vi "Group7.vi"() -> ()   [LabVIEW 2013]
uses:
  Awesome_Statechart.lvsc/StatechartState.ctl
  Awesome_Statechart.lvsc/State.ctl
  <vilib>/myRIO/Instrument Drivers/Onboard IO/DIO/typedefs/DIO Reference.ctl
  <vilib>/myRIO/Common/Instrument Driver Framework/Utilities/typedefs/myRIO Generic Hardware Reference.ctl
  <vilib>/myRIO/Common/Instrument Driver Framework/Utilities/typedefs/Hardware Version Enum.ctl
  <vilib>/myRIO/Common/Instrument Driver Framework/Utilities/typedefs/myRIO v1.0 Reference.ctl
  <vilib>/myRIO/Common/Instrument Driver Framework/Utilities/typedefs/Generic FPGA Reference.ctl
  <vilib>/myRIO/Common/Instrument Driver Framework/myRIO v1.0/DIO/typedefs/DIO Channels List.ctl
  <vilib>/myRIO/Common/Instrument Driver Framework/myRIO v1.0/DIO/typedefs/DIO Channels Enum.ctl
  <vilib>/myRIO/Instrument Drivers/Onboard IO/AI/typedefs/AI Reference.ctl
  <vilib>/myRIO/Common/Instrument Driver Framework/myRIO v1.0/AI/typedefs/AI Channels List.ctl
  <vilib>/myRIO/Common/Instrument Driver Framework/myRIO v1.0/AI/typedefs/AI Channels Enum.ctl
  <vilib>/myRIO/Common/Instrument Driver Framework/Utilities/typedefs/Analog Scaling Constants List.ctl
  <vilib>/myRIO/Common/Instrument Driver Framework/Utilities/typedefs/Analog Scaling Constants.ctl
  <vilib>/myRIO/Instrument Drivers/Onboard IO/PWM/typedefs/PWM Reference.ctl
  <vilib>/myRIO/Common/Instrument Driver Framework/myRIO v1.0/PWM/typedefs/PWM Channels Enum.ctl
  <vilib>/myRIO/Instrument Drivers/Onboard IO/PWM/typedefs/PWM Configuration.ctl
  <vilib>/Platform/TimedLoop/XDataNode/timing_clust.ctl
  <vilib>/Platform/TimedLoop/XDataNode/nitl_modes.ctl
  <vilib>/Platform/TimedLoop/XDataNode/wakeup.ctl
  Awesome_Statechart.lvsc/Inputs.ctl
  Awesome_Statechart.lvsc/CompanionDiagram.vi/38/SC Main.vi
  <vilib>/myRIO/Common/Instrument Driver Framework/myRIO v1.0/PWM/vis/myRIO v1.1 Open PWM.vi
  <vilib>/myRIO/Common/Instrument Driver Framework/myRIO v1.0/AI/vis/myRIO v1.1 Open AI.vi
  <vilib>/myRIO/Common/Instrument Driver Framework/myRIO v1.0/DIO/vis/myRIO v1.1 Open DIO.vi
  Awesome_Statechart.lvsc/CompanionDiagram.vi/38/Upd State.vi
  Awesome_Statechart.lvsc/CompanionDiagram.vi/38/Trans Graph0.vi
  Awesome_Statechart.lvsc/CompanionDiagram.vi/38/EnterGraphCore.vi
  <vilib>/myRIO/Common/Instrument Driver Framework/myRIO v1.0/PWM/vis/myRIO v1.0 Close PWM.vi
  <vilib>/myRIO/Common/Instrument Driver Framework/myRIO v1.0/AI/vis/myRIO v1.0 Close AI.vi
  <vilib>/myRIO/Common/Instrument Driver Framework/myRIO v1.0/DIO/vis/myRIO v1.0 Close DIO.vi
  <vilib>/myRIO/Common/Instrument Driver Framework/Utilities/vis/Validate Channels.vi
  <vilib>/myRIO/Common/Instrument Driver Framework/myRIO v1.0/PWM/vis/myRIO v1.0 Reserve PWM.vi
  <vilib>/myRIO/Common/Instrument Driver Framework/myRIO v1.0/AI/vis/myRIO v1.0 Reserve AI.vi
  <vilib>/myRIO/Common/Instrument Driver Framework/myRIO v1.0/DIO/vis/myRIO v1.0 Reserve DIO.vi
  Awesome_Statechart.lvsc/CompanionDiagram.vi/38/Trans Graph1.vi
  <vilib>/myRIO/Common/Instrument Driver Framework/myRIO v1.0/PWM/vis/myRIO v1.0 Unreserve PWM.vi
  <vilib>/myRIO/Common/Instrument Driver Framework/myRIO v1.0/AI/vis/myRIO v1.0 Unreserve AI.vi
  <vilib>/myRIO/Common/Instrument Driver Framework/myRIO v1.0/DIO/vis/myRIO v1.0 Unreserve DIO.vi
  <vilib>/myRIO/Common/Instrument Driver Framework/myRIO v1.0/PWM/vis/myRIO v1.0 Build MUX Configuration PWM.vi
  <vilib>/myRIO/Common/Instrument Driver Framework/myRIO v1.0/Resource Manager/vis/myRIO v1.0 Reserve Channel List.vi
  <vilib>/myRIO/Common/Instrument Driver Framework/myRIO v1.0/AI/vis/myRIO v1.0 Build MUX Configuration AI.vi
  <vilib>/myRIO/Common/Instrument Driver Framework/myRIO v1.0/DIO/vis/myRIO v1.0 Build MUX Configuration DIO.vi
  Awesome_Statechart.lvsc/CompanionDiagram.vi/38/Trans Graph2.vi
  <vilib>/myRIO/Common/Instrument Driver Framework/myRIO v1.0/Resource Manager/vis/myRIO v1.0 Unreserve Channel List.vi
  <vilib>/myRIO/Common/Instrument Driver Framework/myRIO v1.0/Resource Manager/vis/myRIO v1.0 Create Configuration List.vi
  <vilib>/myRIO/Common/Instrument Driver Framework/myRIO v1.0/Resource Manager/vis/myRIO v1.0 Reserve Channel.vi
  <vilib>/myRIO/Common/Instrument Driver Framework/myRIO v1.0/Resource Manager/vis/myRIO v1.0 Unreserve Channel.vi
  <vilib>/myRIO/Common/Instrument Driver Framework/myRIO v1.0/Resource Manager/vis/myRIO v1.0 Build Mutex Name.vi
  <vilib>/FPGAPlugInAG/myRIO-1900/niLvFpga_Open_myRIO-1900.vi
  <vilib>/rvi/interface/common/dynamic/niFpgaDynamicAddResources.vi
  <vilib>/myRIO/Common/Instrument Driver Framework/Utilities/vis/FPGA Ref Manager.vi
  <vilib>/Utility/error.llb/Error Cluster From Error Code.vi
  <vilib>/rvi/interface/common/niFpgaWaitOnOcc.vi
  <vilib>/myRIO/Common/Instrument Driver Framework/myRIO v1.0/myRIO v1.1 Open.vi
  <vilib>/Utility/VariantDataType/GetNumericInfo.vi
  <vilib>/myRIO/Common/Instrument Driver Framework/Utilities/vis/IO Manager.vi
  <vilib>/myRIO/Common/Instrument Driver Framework/Utilities/vis/Configuration Manager.vi
  <vilib>/myRIO/Common/Instrument Driver Framework/myRIO v1.0/Resource Manager/vis/myRIO v1.0 Configure IO.vi
  <vilib>/myRIO/Common/Instrument Driver Framework/myRIO v1.0/myRIO v1.0 Close.vi
  <vilib>/myRIO/Common/Instrument Driver Framework/myRIO v1.0/AI/vis/myRIO v1.0 Get Scaling Constants AI.vi
  <vilib>/myRIO/Common/Instrument Driver Framework/myRIO v1.0/DIO/vis/myRIO v1.0 Read DIO.vi
  <vilib>/myRIO/Common/Instrument Driver Framework/myRIO v1.0/DIO/vis/myRIO v1.0 Write DIO.vi
  <vilib>/myRIO/Common/Instrument Driver Framework/myRIO v1.0/PWM/vis/myRIO v1.0 Write PWM.vi
  <vilib>/myRIO/Common/Instrument Driver Framework/myRIO v1.0/AI/vis/myRIO v1.0 Read AI.vi
  Awesome_Statechart.lvsc/CompanionDiagram.vi
  <vilib>/rvi/errors/niLvFpgaAdjustHostInterfaceError.vi
  <vilib>/myRIO/Common/Instrument Driver Framework/myRIO v1.0/DIO/vis/myRIO v1.0 Shutdown DIO.vi
  <vilib>/myRIO/Common/Instrument Driver Framework/myRIO v1.0/PWM/vis/myRIO v1.0 Shutdown PWM.vi
  <vilib>/FPGAPlugInAG/Dynamic/niLvFpga_Close_Dynamic.vi
  <vilib>/rvi/interface/nirviOpenFPGA/nirviOpenFPGA.xnode
  FPGA Bitfiles/MAE162Labs_FPGATarget_myRIO-1900Custom_wGhQFU+VMJc.lvbitx
  <vilib>/rvi/interface/nirviMethod/nirviMethod.xnode
  <vilib>/Platform/TimedLoop/XDataNode/XDataNode.xnode
  Awesome_Statechart.lvsc/Trigger.ctl
  <vilib>/Statechart/Infrastructure/RTStatechart/RunTime SCN.xnode
  Awesome_Statechart.lvsc/Outputs.ctl
  Awesome_Statechart.lvsc
  <vilib>/rvi/interface/nirviCloseFPGA/nirviCloseFPGA.xnode
  <vilib>/Platform/TimedLoop/XDataNode/XDNodeRunTimeDep.lvlib
  <vilib>/rvi/interface/nirviMethod/StockFPGA_InlinedMethodWaitForSingleIRQ.vi
  <vilib>/FPGAPlugInAG/Dynamic/niLvFpga_WaitOnIrq_Dynamic.vi
  <vilib>/FPGAPlugInAG/Dynamic/niLvFpga_AcknowledgeIrq_Dynamic.vi
  <vilib>/myRIO/Instrument Drivers/Utilities/Utilities.lvlib
  <vilib>/myRIO/Instrument Drivers/Onboard IO/DIO/DIO.lvlib
  <vilib>/myRIO/Instrument Drivers/Onboard IO/AI/AI.lvlib
  <vilib>/myRIO/Instrument Drivers/Onboard IO/PWM/PWM.lvlib
panel:
  in  "Pulse Width":dbl=2280.0
  out "Left Duty Cycle":dbl(graph)
  out "Right Duty Cycle":dbl(graph)
  in  "moving up ramp gains":cluster{"Kp":dbl, "Kd":dbl, "Ki":dbl, "Ts":dbl}={"Kp"=0.01, "Kd"=0.0, "Ki"=0.008, "Ts"=0.01}
  out "duty 2":dbl=0.012080000000000046
  in  "Gain Mode 2":dbl=2.5
  out "PID Output 2":dbl=0.004832000000000019
  out "L_DC 2":dbl=-0.38308
  out "R_DC 2":dbl=-0.41692000000000007
  in  "Reverse?":bool
  in  "Default_Speed":dbl=0.4
  in  "On Ramp?":bool
  out "WindUp Servo":i16=1525
  out "R_DC":dbl=0.06510400000000012
  out "L_DC":dbl=-0.06510400000000012
  out "Moving Up Ramp?":bool
  out "Finding Entrance?":bool
  out "PID Output":dbl=0.03272000000000006
  out "R_DC_STATE":dbl
  out "L_DC_STATE":dbl
  out "duty":dbl=0.06544000000000012
  in  "Gain Mode 1":dbl=2.0
  in  "moving down ramp gainz":cluster{"Kp":dbl, "Kd":dbl, "Ki":dbl, "Ts":dbl}={"Kp"=0.02, "Kd"=0.0, "Ki"=0.016, "Ts"=0.01}
  out "Mode":i16=3
  in  "BLACK BOX GRAPH":enum32{"Page 1", "Page 2", "Page 3"}(tab)=enum."Page 2"
  out "Black Box":T1(graph)
  out "Black Box Array":dbl[][](array[numeric])
  out "Array":bool[](array[boolean])
  out "Button Num":u32
  in  "ON":bool
  in  "OFF":bool
  out "Active States":T2=[enum."On", enum."On\\Region\\Running"]
  out "Front Right":dbl=6.1
  out "Front Left":dbl=7.5
  out "Back Right":dbl=7.6
  out "Center":dbl=6.692913385826771
  out "Back Left":dbl=7.9
  out "Finished Late":u16
  out "Emergency Stop":bool=TRUE
  # "1000 to 2000; 1500 max"
  # "Coming Out of Statechart"
  # "2000 max"
  # "800 max"
  # "MOVING DOWN RAMP"
  # "MOVING UP RAMP"
  # "Coming Out of PID"
  # "3rd bin: 2280\n2nd bin: 2150\n1st bin: 1950"
  # "After Calculations"
  # "SENSORS"
  # "gAIN = 2"
  # "MOTORS"
  # "KP=0.02"
  # "moving up:\nKp = 0.01\nki = 0.008\n\nts = 0.01\n\nmoving down:\nkp = 0.02\nki = 0.016\nts = 0.01"
  # "0: Find Entrance\n1: Move Up\n2: Move Down\n3: Default"
  # "SERVOS"
  # "kI = 0.016"
  # "NOTE: Continuous Servo Mid-Point = 1525\nPlatform Servo Mid-Point = 1500"
  # "tS = 0.01"
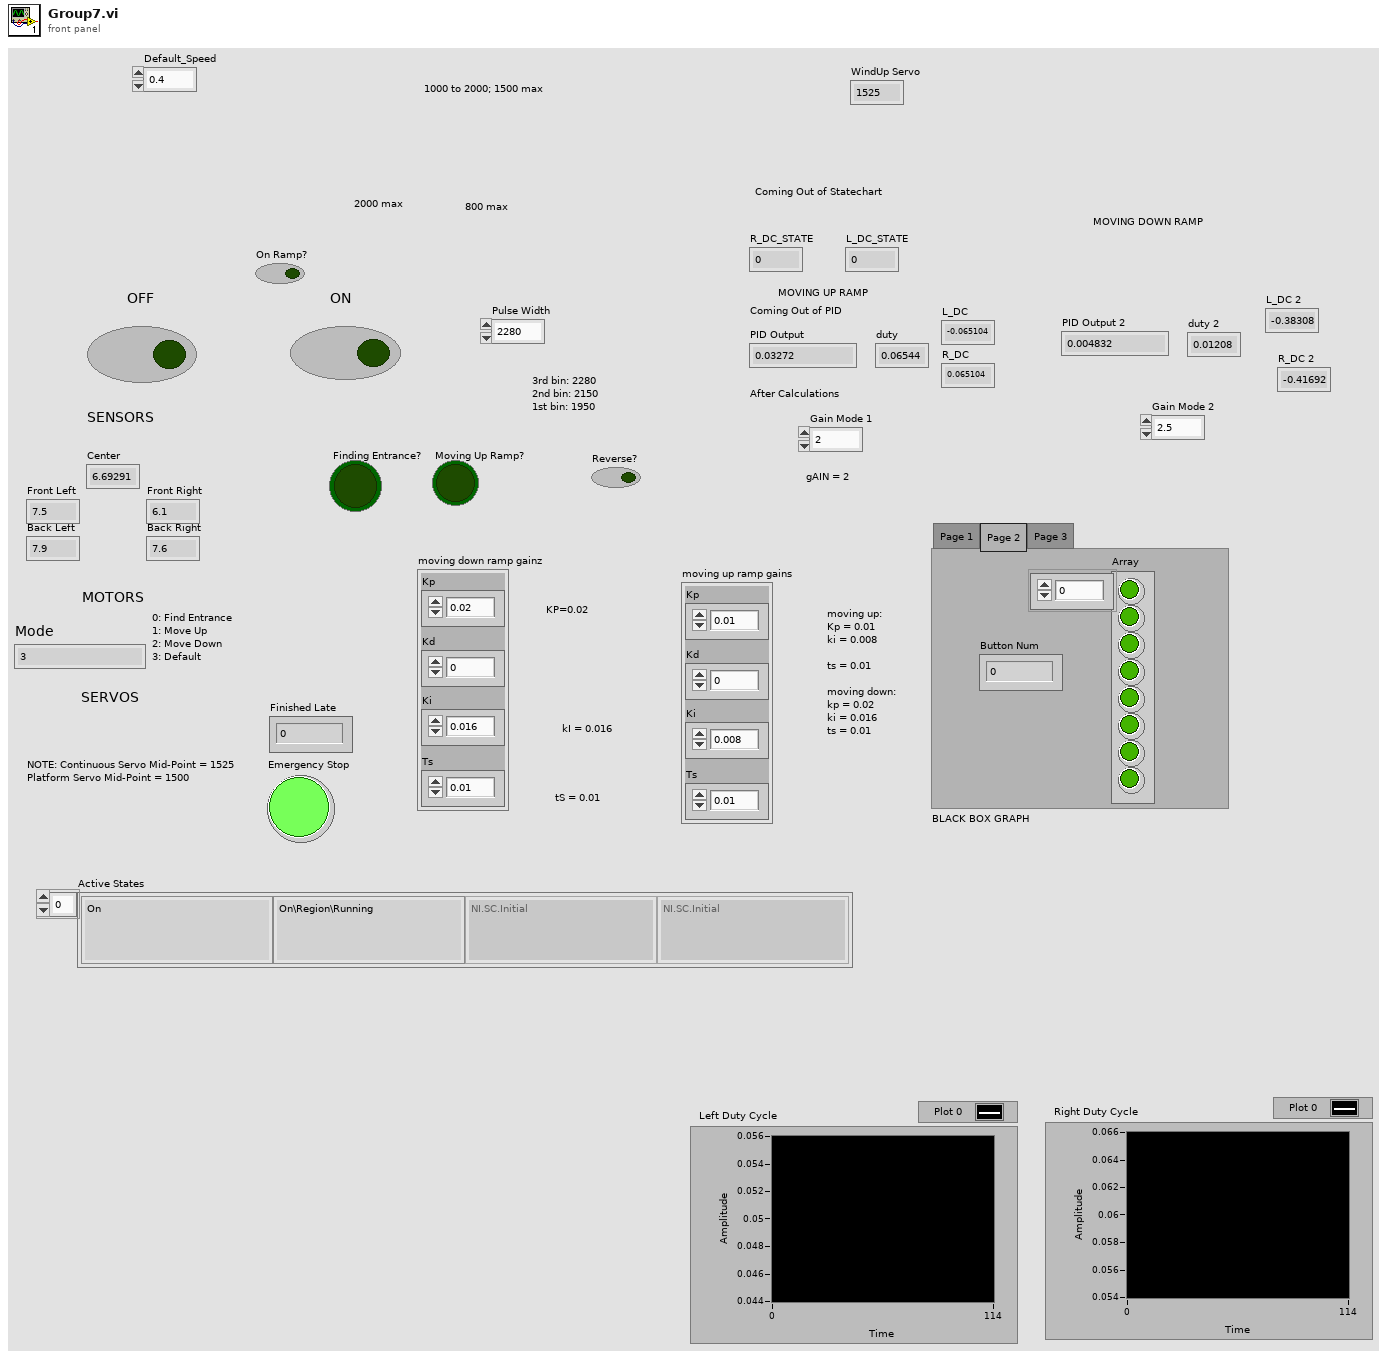
[diagram p1: front panel]
types:
  T1 = cluster{"[0]":dbl, "[1]":dbl, "[2]":dbl, "[3]":dbl, "[4]":dbl, "[5]":dbl, "[6]":dbl, "[7]":dbl}
  T2 = typedef "Awesome_Statechart.lvsc/StatechartState.ctl" = T3[]
  T3 = typedef "Awesome_Statechart.lvsc/State.ctl" = enum16{"NI.SC.Initial", "NI.SC.History", "NI.SC.ShallowHistory", "NI.SC.Terminal", "On", "Off", "On\\Region\\Straighten", "On\\Region\\Wait", "On\\Region\\Fire Cannon", "On\\Region\\Moving Down Ramp", "On\\Region\\Moving Up Ramp", "On\\Region\\Find_Entrance", "On\\Region\\Running", "On\\Region\\Find_Entrance\\Region\\Entrance\nOn\nRight Side", "On\\Region\\Find_Entrance\\Region\\Entrance \nOn\nLeft Side", "On\\Region\\Find_Entrance\\Region\\Turn Right", "On\\Region\\Find_Entrance\\Region\\Turn Left", "On\\Region\\Find_Entrance\\Region\\Go_Straight", "On\\Region\\Find_Entrance\\Region\\Running"}
  T4 = typedef "DIO.lvlib/DIO Reference.ctl" = cluster{"myRIO Reference":T5, "DIO Channels List":T9}
  T5 = typedef "myRIO Generic Hardware Reference.ctl" = cluster{"myRIO Model":T6, "myRIO Hardware Reference":T7}
  T6 = typedef "Hardware Version Enum.ctl" = enum16{"Unknown", "myRIO-1900", "myRIO-1950"}
  T7 = typedef "myRIO v1.0 Reference.ctl" = cluster{"Generic FPGA Reference":T8, "Allow multiple opens":bool}
  T8 = typedef "Generic FPGA Reference.ctl" = refnum<k20>
  T9 = typedef "DIO Channels List.ctl" = T10[]
  T10 = typedef "DIO Channels Enum.ctl" = enum16{"Not Connected", "C/DIO0", "C/DIO1", "C/DIO2", "C/DIO3", "C/DIO4", "C/DIO5", "C/DIO6", "C/DIO7", "A/DIO0", "A/DIO1", "A/DIO2", "A/DIO3", "A/DIO4", "A/DIO5", "A/DIO6", "A/DIO7", "A/DIO8", "A/DIO9", "A/DIO10", "A/DIO11", "A/DIO12", "A/DIO13", "A/DIO14", "A/DIO15", "B/DIO0", "B/DIO1", "B/DIO2", "B/DIO3", "B/DIO4", "B/DIO5", "B/DIO6", "B/DIO7", "B/DIO8", "B/DIO9", "B/DIO10", "B/DIO11", "B/DIO12", "B/DIO13", "B/DIO14", "B/DIO15", "LED0", "LED1", "LED2", "LED3", "Button0"}
  T11 = typedef "AI.lvlib/AI Reference.ctl" = cluster{"myRIO Reference":T5, "AI Channels List":T12, "AI Scaling Constants List":T14}
  T12 = typedef "AI Channels List.ctl" = T13[]
  T13 = typedef "AI Channels Enum.ctl" = enum16{"Not Connected", "AudioIn/Left", "AudioIn/Right", "C/AI0", "C/AI1", "A/AI0", "A/AI1", "A/AI2", "A/AI3", "B/AI0", "B/AI1", "B/AI2", "B/AI3"}
  T14 = typedef "Analog Scaling Constants List.ctl" = T15[]
  T15 = typedef "Analog Scaling Constants.ctl" = cluster{"LSB Weight (Volts)":dbl, "Offset (Volts)":dbl, "Signed?":bool}
  T16 = typedef "PWM.lvlib/PWM Reference.ctl" = cluster{"myRIO Reference":T5, "PWM Channels Enum":T17, "PWM Configuration":T18}
  T17 = typedef "PWM Channels Enum.ctl" = enum16{"Not Connected", "C/PWM0", "C/PWM1", "A/PWM0", "A/PWM1", "A/PWM2", "B/PWM0", "B/PWM1", "B/PWM2"}
  T18 = typedef "PWM.lvlib/PWM Configuration.ctl" = cluster{"Frequency":dbl, "Duty Cycle":dbl}
  T19 = cluster{"Button Ref":T4, "LED Ref":T4, "Front_Right":T11, "Front_Left":T11, "Back_Right":T11, "Front_Center\nBI Ref 1":T11, "Back_Left\nBI Ref 2":T11, "Windup":T16, "Platform_S\nPlatform_S\nContinuous Servo":T16, "Left Motor\nLeft Motor\nright_motor":T16, "Right Motor\nleft_motor":T16}
  T20 = typedef "XDNodeRunTimeDep.lvlib/timing_clust.ctl" = cluster{"Expected End [f-1]":u64, "Actual End [f-1]":u64, "Finished Late? [f-1]":bool, "Expected End [i-1]":u64, "Actual End [i-1]":u64, "Finished Late? [i-1]":bool, "Expected Start [i]":u64, "Actual Start [i]":u64, "Expected Start [f]":u64, "Actual Start [f]":u64, "Source Name":string, "Structure Name":string, "Period":i64, "Deadline":i64, "Offset":i64, "Start":i64, "Priority":i32, "Timeout":i32, "Mode":T21, "Wakeup Reason":T22, "Error":errorcluster, "Source Type":string, "Secondary Source Type":string, "Global End Time":u64, "Global Start Time":u64, "Frame Duration":u64, "Iteration Duration":u64, "Assigned CPU":i32, "I/O Scan Engine Mode":u32}
  T21 = typedef "XDNodeRunTimeDep.lvlib/nitl_modes.ctl" = enum32{"No Change", "Process missed periods, maintain original phase", "Discard missed periods, maintain original phase", "Process missed periods, ignore original phase", "Discard missed periods, ignore original phase"}
  T22 = typedef "XDNodeRunTimeDep.lvlib/wakeup.ctl" = enum32{"Normal", "Aborted", "Asynchronous wakeup", "Timing source error", "Timed loop error", "Timeout"}
  T23 = typedef "Awesome_Statechart.lvsc/Inputs.ctl" = cluster{"On/Set":bool, "Off":bool, "Front_Center ":dbl, "Front_Left":dbl, "Front_Right":dbl, "Back_Left":dbl, "Back_Right":dbl, "Find_Entrance?":bool, "Default_Speed":dbl, "On Ramp?":bool, "Bombs Away!":bool, "Reverse?":bool}
  T24 = typedef "Awesome_Statechart.lvsc/Outputs.ctl" = cluster{"Left_Duty":dbl, "Right_Duty":dbl, "Mode":i16, "Finding Entrance?":bool, "Moving Up Ramp?":bool, "WindUp Servo":i16, "Straighten?":bool, "Platform Servo":dbl}
  T25 = cluster{"[0]":dbl, "[1]":dbl, "[2]":dbl, "[3]":dbl, "[4]":dbl, "[5]":dbl, "[6]":dbl, "[7]":dbl}[]
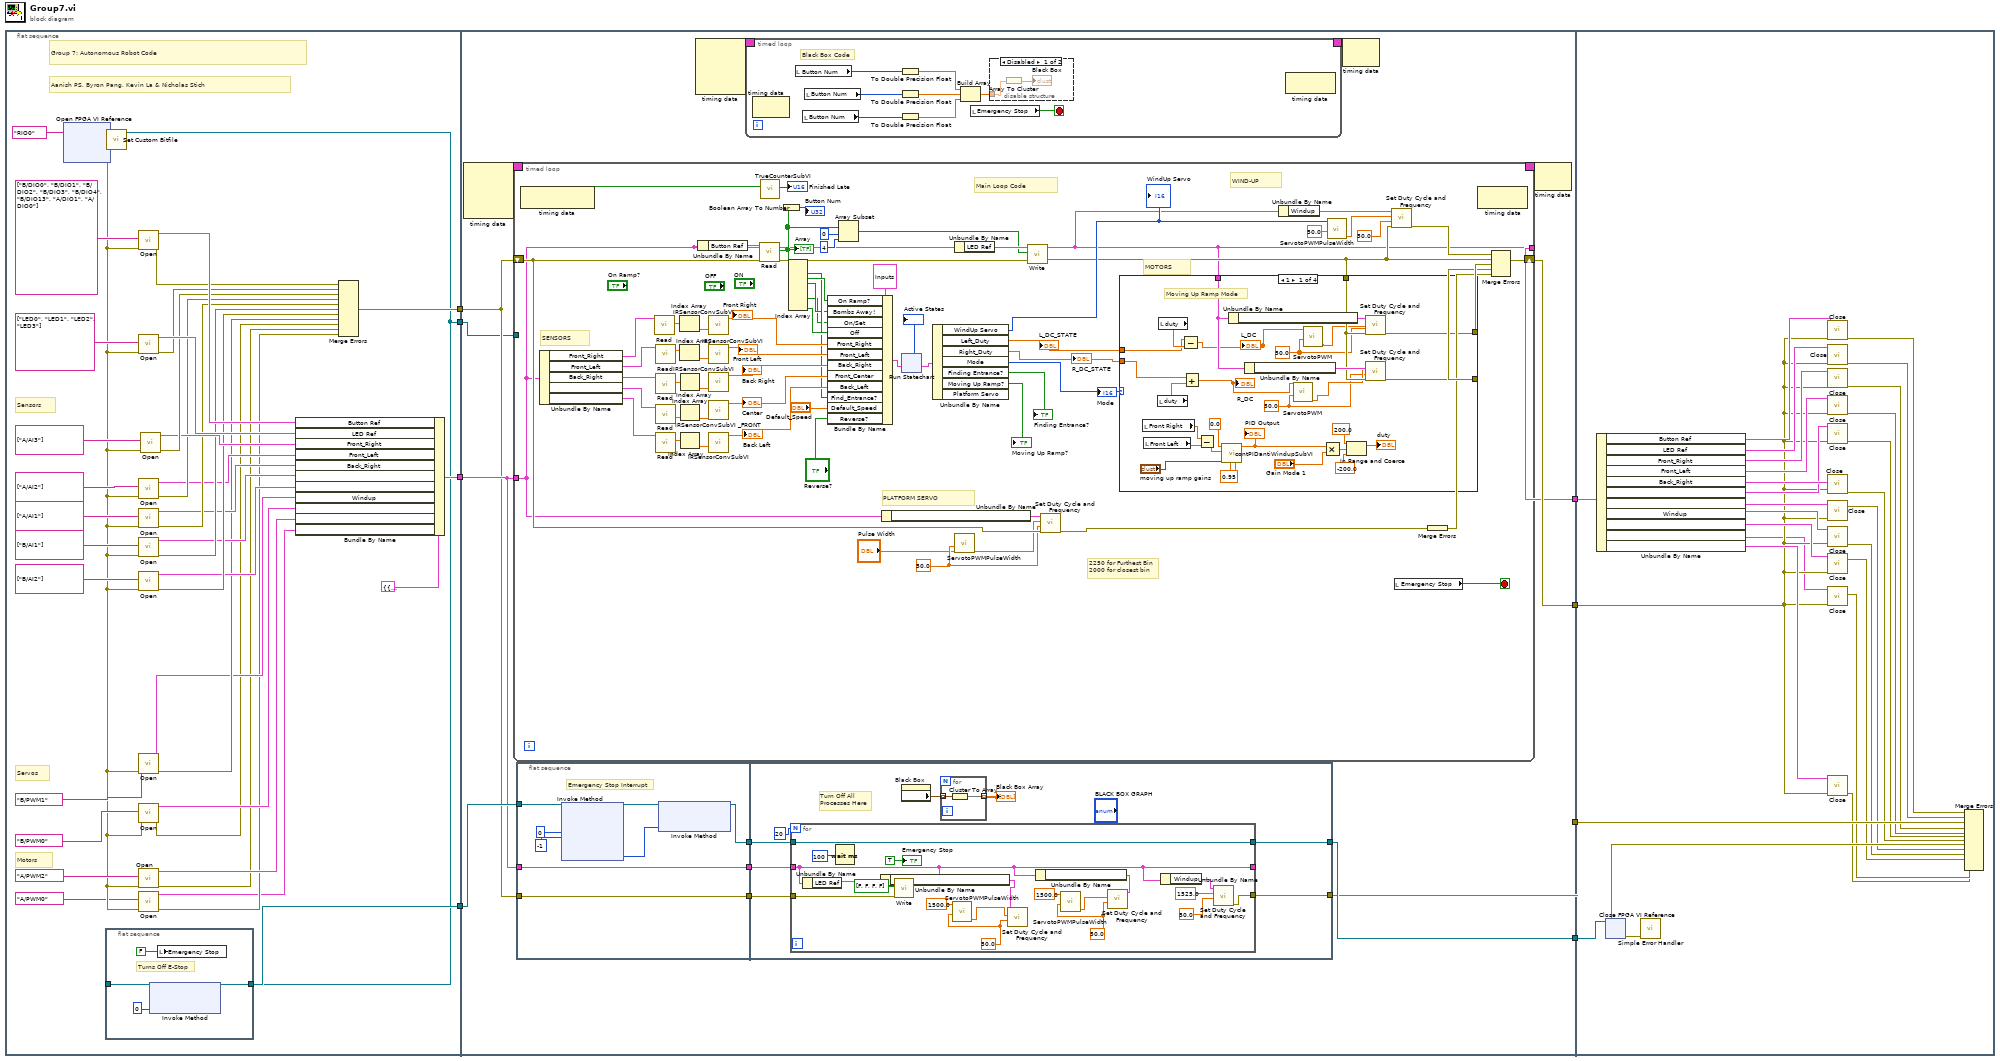
[diagram p0: block diagram]
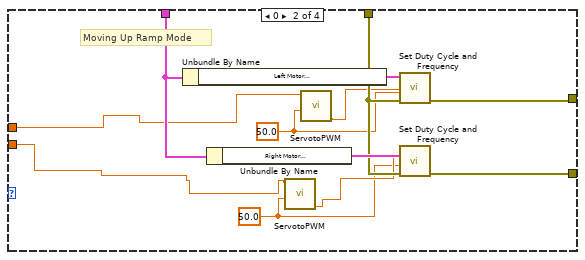
[diagram p3: hidden frame]
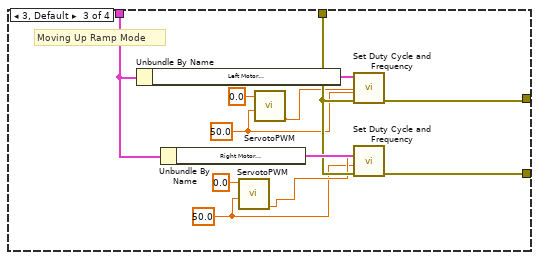
[diagram p4: hidden frame]
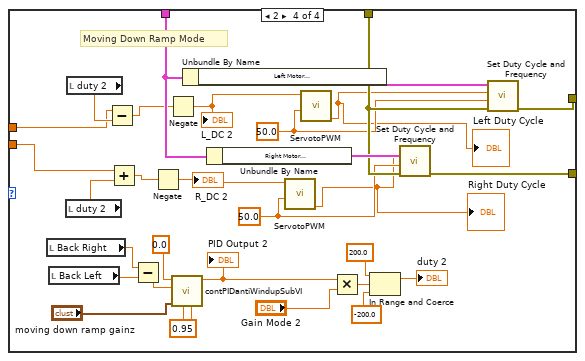
[diagram p5: hidden frame]
diagram:
  n1 = flat-sequence {
    tunnel: [w50] -> w8
    tunnel: [w40] -> w6
    tunnel: [w39] -> w5
    tunnel: [w38] -> w1
    tunnel: [w64] -> w7
    tunnel: w8 -> [w63]
    tunnel: w6 -> [w62]
    tunnel: w5 -> [w59]
    tunnel: [w58] -> w4
    tunnel: [w55] -> w3
    tunnel: [w57] -> w2
    tunnel: w1 -> [w56]
    tunnel: w7 -> [w405]
    tunnel: w4 -> [w379]
    tunnel: w3 -> [w404]
    tunnel: w2 -> [w397]
    frame #0 {
      # "Aanish PS, Byron Pang, Kevin La & Nicholas Stich"
      # "Group 7: Autonomous Robot Code"
      # "Servos"
      # "Motors"
      # "Sensors"
      n2 = xnode "Open FPGA VI Reference"("resource name"=tag "RIO0") -> ("FPGA VI Reference Out"=w49:refnum<k20>, "error out"=w48:errorcluster)  [unwired: 1 in]
      n3 = flat-sequence {
        tunnel: [w52] -> w50
        tunnel: w38 -> [w53]
        frame #0 {
          # "Turns Off E-Stop"
          n4 = xnode "Invoke Method"("FPGA VI Reference In"=w53, "IRQ Number(s)"=0) -> ("FPGA VI Reference Out"=w52:refnum<k20>)  [unwired: 1 in, 1 out]
          n5 = local write "Emergency Stop"(FALSE ("Emergency Stop")) -> ()
        }
      }
      n6 = call <vilib>:"Set Custom Bitfile.vi"("error in (no error)"=w48, "Customized FPGA Reference in"=w49) -> ("error out"=w15:errorcluster, "Customized FPGA Reference out"=w38:refnum<k20>)  [unwired: 8 in]
      n7 = call <vilib>:"Open.vi"("error in (no error)"=w15, "Channel Names"=tag[] ["B/DIO0", "B/DIO1", "B/DIO2", "B/DIO3", "B/DIO4", "B/DIO13", "A/DIO1", "A/DIO0"]) -> ("error out"=w42:errorcluster, "DIO Ref Out"=w44:T4)  [unwired: 8 in]
      n8 = call <vilib>:"Open.vi"("error in (no error)"=w15, "Channel Names"=tag[] ["LED0", "LED1", "LED2", "LED3"]) -> ("error out"=w41:errorcluster, "DIO Ref Out"=w43:T4)  [unwired: 8 in]
      n9 = call <vilib>:"Open.vi"("error in (no error)"=w15, "Channel Names"=tag[] ["A/AI2"]) -> ("error out"=w32:errorcluster, "AI Ref Out"=w26:T11)  [unwired: 8 in]
      n10 = call <vilib>:"Open.vi"("error in (no error)"=w15, "Channel Names"=tag[] ["A/AI1"]) -> ("error out"=w31:errorcluster, "AI Ref Out"=w25:T11)  [unwired: 8 in]
      n11 = call <vilib>:"Open.vi"("error in (no error)"=w15, "Channel Names"=tag[] ["B/AI1"]) -> ("error out"=w29:errorcluster, "AI Ref Out"=w24:T11)  [unwired: 8 in]
      n12 = call <vilib>:"Open.vi"("error in (no error)"=w15, "Channel Names"=tag[] ["B/AI2"]) -> ("error out"=w27:errorcluster, "AI Ref Out"=w23:T11)  [unwired: 8 in]
      n13 = call <vilib>:"Open.vi"("error in (no error)"=w15, "Channel Name"=tag "B/PWM1") -> ("error out"=w21:errorcluster, "PWM Ref Out"=w20:T16)  [unwired: 8 in]
      n14 = call <vilib>:"Open.vi"("error in (no error)"=w15, "Channel Name"=tag "B/PWM0") -> ("error out"=w11:errorcluster, "PWM Ref Out"=w18:T16)  [unwired: 8 in]
      n15 = call <vilib>:"Open.vi"("error in (no error)"=w15, "Channel Name"=tag "A/PWM2") -> ("error out"=w10:errorcluster, "PWM Ref Out"=w16:T16)  [unwired: 8 in]
      n16 = call <vilib>:"Open.vi"("error in (no error)"=w15, "Channel Name"=tag "A/PWM0") -> ("error out"=w13:errorcluster, "PWM Ref Out"=w12:T16)  [unwired: 8 in]
      n17 = call <vilib>:"Open.vi"("error in (no error)"=w15, "Channel Names"=tag[] ["A/AI3"]) -> ("error out"=w37:errorcluster, "AI Ref Out"=w36:T11)  [unwired: 8 in]
      n18 = Bundle By Name(cluster=T19 {"Button Ref"={"myRIO Reference"={"myRIO Model"=enum."Unknown", "myRIO Hardware Reference"={"Generic FPGA Reference"=refnum, "Allow multiple opens"=FALSE}}, "DIO Channels List"=[]}, "LED Ref"={"myRIO Reference"={"myRIO Model"=enum."Unknown", "myRIO Hardware Reference"={"Generic FPGA Reference"=refnum, "Allow multiple opens"=FALSE}}, "DIO Channels List"=[]}, "Front_Right"={"myRIO Reference"={"myRIO Model"=enum."Unknown", "myRIO Hardware Reference"={"Generic FPGA Reference"=refnum, "Allow multiple opens"=FALSE}}, "AI Channels List"=[], "AI Scaling Constants List"=[]}, "Front_Left"={"myRIO Reference"={"myRIO Model"=enum."Unknown", "myRIO Hardware Reference"={"Generic FPGA Reference"=refnum, "Allow multiple opens"=FALSE}}, "AI Channels List"=[], "AI Scaling Constants List"=[]}, "Back_Right"={"myRIO Reference"={"myRIO Model"=enum."Unknown", "myRIO Hardware Reference"={"Generic FPGA Reference"=refnum, "Allow multiple opens"=FALSE}}, "AI Channels List"=[], "AI Scaling Constants List"=[]}, "Front_Center\nBI Ref 1"={"myRIO Reference"={"myRIO Model"=enum."Unknown", "myRIO Hardware Reference"={"Generic FPGA Reference"=refnum, "Allow multiple opens"=FALSE}}, "AI Channels List"=[], "AI Scaling Constants List"=[]}, "Back_Left\nBI Ref 2"={"myRIO Reference"={"myRIO Model"=enum."Unknown", "myRIO Hardware Reference"={"Generic FPGA Reference"=refnum, "Allow multiple opens"=FALSE}}, "AI Channels List"=[], "AI Scaling Constants List"=[]}, "Windup"={"myRIO Reference"={"myRIO Model"=enum."Unknown", "myRIO Hardware Reference"={"Generic FPGA Reference"=refnum, "Allow multiple opens"=FALSE}}, "PWM Channels Enum"=enum."Not Connected", "PWM Configuration"={"Frequency"=0.0, "Duty Cycle"=0.0}}, "Platform_S\nPlatform_S\nContinuous Servo"={"myRIO Reference"={"myRIO Model"=enum."Unknown", "myRIO Hardware Reference"={"Generic FPGA Reference"=refnum, "Allow multiple opens"=FALSE}}, "PWM Channels Enum"=enum."Not Connected", "PWM Configuration"={"Frequency"=0.0, "Duty Cycle"=0.0}}, "Left Motor\nLeft Motor\nright_motor"={"myRIO Reference"={"myRIO Model"=enum."Unknown", "myRIO Hardware Reference"={"Generic FPGA Reference"=refnum, "Allow multiple opens"=FALSE}}, "PWM Channels Enum"=enum."Not Connected", "PWM Configuration"={"Frequency"=0.0, "Duty Cycle"=0.0}}, "Right Motor\nleft_motor"={"myRIO Reference"={"myRIO Model"=enum."Unknown", "myRIO Hardware Reference"={"Generic FPGA Reference"=refnum, "Allow multiple opens"=FALSE}}, "PWM Channels Enum"=enum."Not Connected", "PWM Configuration"={"Frequency"=0.0, "Duty Cycle"=0.0}}}, "Button Ref"=w44, "LED Ref"=w43, "Front_Right"=w36, "Front_Left"=w26, "Back_Right"=w25, "Front_Center\nBI Ref 1"=w24, "Back_Left\nBI Ref 2"=w23, "Windup"=w20, "Platform_S\nPlatform_S\nContinuous Servo"=w18, "Left Motor\nLeft Motor\nright_motor"=w16, "Right Motor\nleft_motor"=w12) -> (w40:T19)
      n19 = Merge Errors(w42, w41, w37, w32, w31, w29, w27, w21, w11, w10, w13) -> (w39:errorcluster)
    }
    frame #1 {
      n20 = node-c288() -> (w69:T20)  [unwired: 4 in]
      n21 = timed-loop {
        timing: w69 -> [_]
        timing-out: [_] -> w68
        tunnel: w62 -> [w134]
        tunnel: [w134] -> w55
        shift-right: [w161] -> w58
        shift-left: w59 -> [w139]
        tunnel: w56 -> [_]
        stop <- w185 stop-if-true
        w124 = 50.0 ("Frequency (Hz)")
        # "PLATFORM SERVO"
        # "MOTORS"
        # "2250 for Furthest Bin\n2000 for closest bin"
        # "WIND-UP"
        # "SENSORS"
        # "Main Loop Code"
        n22 = node-c288() -> (w183:bool)  [unwired: 1 in]
        n23 = Unbundle By Name(w134) -> ("Front_Right"=w162:T11, "Front_Left"=w163:T11, "Back_Right"=w156:T11, "Front_Center\nBI Ref 1"=w164:T11, "Back_Left\nBI Ref 2"=w165:T11)
        n24 = call <vilib>:"Read.vi"("AI Ref In"=w162) -> ("Values"=w175:dbl[])  [unwired: 8 in, 2 out]
        n25 = call <vilib>:"Read.vi"("AI Ref In"=w163) -> ("Values"=w174:dbl[])  [unwired: 8 in, 2 out]
        n26 = call <vilib>:"Read.vi"("AI Ref In"=w156) -> ("Values"=w173:dbl[])  [unwired: 8 in, 2 out]
        n27 = call <vilib>:"Read.vi"("AI Ref In"=w164) -> ("Values"=w172:dbl[])  [unwired: 8 in, 2 out]
        n28 = call <vilib>:"Read.vi"("AI Ref In"=w165) -> ("Values"=w171:dbl[])  [unwired: 8 in, 2 out]
        n29 = Index Array(array=w175) -> (element=w170:dbl)  [unwired: 1 in]
        n30 = Index Array(array=w174) -> (element=w167:dbl)  [unwired: 1 in]
        n31 = Index Array(array=w173) -> (element=w168:dbl)  [unwired: 1 in]
        n32 = Index Array(array=w172) -> (element=w166:dbl)  [unwired: 1 in]
        n33 = Index Array(array=w171) -> (element=w169:dbl)  [unwired: 1 in]
        n34 = Unbundle By Name(w134) -> ("Button Ref"=w179:T4)
        n35 = call "IRSensorConvSubVI.vi"("Infrared Sensor Reading"=w170) -> ("Sensor Data"=w152:dbl)  [unwired: 10 in]
        "Front Right" <- w152
        n36 = call "IRSensorConvSubVI.vi"("Infrared Sensor Reading"=w167) -> ("Sensor Data"=w149:dbl)  [unwired: 10 in]
        "Front Left" <- w149
        n37 = call "IRSensorConvSubVI.vi"("Infrared Sensor Reading"=w168) -> ("Sensor Data"=w155:dbl)  [unwired: 10 in]
        "Back Right" <- w155
        n38 = call "IRSensorConvSubVI _FRONT.vi"("Infrared Sensor Reading"=w166) -> ("Sensor Data"=w154:dbl)  [unwired: 10 in]
        "Center" <- w154
        n39 = call "IRSensorConvSubVI.vi"("Infrared Sensor Reading"=w169) -> ("Sensor Data"=w153:dbl)  [unwired: 10 in]
        "Back Left" <- w153
        n40 = call <vilib>:"Read.vi"("error in (no error)"=w139, "DIO Ref In"=w179) -> ("error out"=w178:errorcluster, "Values"=w145:bool[])  [unwired: 7 in, 1 out]
        "Array" <- w145
        n41 = call "TrueCounterSubVI.vi"("True?"=w183) -> ("True Count"=→"Finished Late":u16)  [unwired: 9 in]
        n42 = Boolean Array To Number(Boolean array=w145) -> (number=→"Button Num":u32)
        n43 = Index Array(array=w145) -> (element #1=w128:bool, element #2=w132:bool, element #3=w127:bool, element #6=w126:bool, element #8=w129:bool)  [unwired: 8 in, 3 out]
        n44 = Bundle By Name(cluster=T23 {"On/Set"=FALSE, "Off"=FALSE, "Front_Center "=0.0, "Front_Left"=0.0, "Front_Right"=0.0, "Back_Left"=0.0, "Back_Right"=0.0, "Find_Entrance?"=FALSE, "Default_Speed"=0.0, "On Ramp?"=FALSE, "Bombs Away!"=FALSE, "Reverse?"=FALSE} ("Inputs"), "On Ramp?"=w132, "Bombs Away!"=w127, "On/Set"=w126, "Off"=w129, "Front_Right"=w152, "Front_Left"=w149, "Back_Right"=w155, "Front_Center"=w154, "Back_Left"=w153, "Find_Entrance?"=w128, "Default_Speed"="Default_Speed", "Reverse?"="Reverse?") -> (w159:T23)
        n45 = Array Subset(array=w145, index=0, length=4) -> (w176:bool[])
        n46 = Unbundle By Name(w134) -> ("Platform_S\nPlatform_S\nContinuous Servo"=w123:T16)
        n47 = xnode "Run Statechart"("Inputs"=w159) -> ("Outputs"=w157:T24, "Active States"=→"Active States":T2)  [unwired: 2 in, 1 out]
        n48 = Unbundle By Name(w157) -> ("WindUp Servo"=w142:i16, "Left_Duty"=w147:dbl, "Right_Duty"=w148:dbl, "Mode"=w146:i16, "Finding Entrance?"=→"Finding Entrance?":bool, "Moving Up Ramp?"=→"Moving Up Ramp?":bool)  [unwired: 1 out]
        "Mode" <- w146
        "L_DC_STATE" <- w147
        "R_DC_STATE" <- w148
        "WindUp Servo" <- w142
        n49 = Unbundle By Name(w134) -> ("LED Ref"=w177:T4)
        n50 = call "ServotoPWMPulseWidth.vi"("freq [Hz]"=w124, "Pulse Width"="Pulse Width") -> ("Duty Cycle"=w122:dbl)  [unwired: 6 in, 2 out]
        n51 = call <vilib>:"Write.vi"("error in (no error)"=w178, "Values"=w176, "DIO Ref In"=w177) -> ("error out"=w140:errorcluster)  [unwired: 6 in, 1 out]
        n52 = call <vilib>:"Set Duty Cycle and Frequency.vi"("error in (no error)"=w139, "Frequency (Hz)"=w124, "Duty Cycle (0-1)"=w122, "PWM Ref In"=w123) -> ("error out"=w125:errorcluster)  [unwired: 5 in, 1 out]
        n53 = case shown="1" w146 {
          tunnel: w134 -> [w213 w225 w237 w267]
          tunnel: [w210 w222 w234 w264] -> w151
          tunnel: [w209 w221 w233 w263] -> w150
          tunnel: w148 -> [w195 w214 _ w249]
          tunnel: w147 -> [w193 w215 _ w247]
          tunnel: w140 -> [w198 w220 w232 w252]
          frame 1 {
            w200 = 0.95 ("Saturation U")
            w189 = 50.0 ("freq [Hz]")
            w191 = 50.0 ("freq [Hz]")
            # "Moving Up Ramp Mode"
            n54 = local read "Front Right"() -> (w207:dbl)
            n55 = local read "Front Left"() -> (w205:dbl)
            n56 = local read "duty"() -> (w196:dbl)
            n57 = local read "duty"() -> (w194:dbl)
            n58 = Subtract(x=w193, y=w194) -> (x-y=w187:dbl)
            "L_DC" <- w187
            n59 = Add(x=w195, y=w196) -> (x+y=w188:dbl)
            "R_DC" <- w188
            n60 = Subtract(x=w207, y=w205) -> (x-y=w206:dbl)
            n61 = call "contPIDantiWindupSubVI.vi"("Saturation M"=w200, "Saturation U"=w200, "PID Gains"="moving up ramp gains", "Position"=w206, "Reference"=0.0) -> ("control"=w197:dbl)  [unwired: 6 in]
            "PID Output" <- w197
            n62 = Unbundle By Name(w213) -> ("Left Motor\nLeft Motor\nright_motor"=w212:T16)
            n63 = Unbundle By Name(w213) -> ("Right Motor\nleft_motor"=w211:T16)
            n64 = call "ServotoPWM.vi"("freq [Hz]"=w189, "Duty In"=w188) -> ("Duty Cycle"=w190:dbl)  [unwired: 6 in, 2 out]
            n65 = call "ServotoPWM.vi"("freq [Hz]"=w191, "Duty In"=w187) -> ("Duty Cycle"=w192:dbl)  [unwired: 6 in, 2 out]
            n66 = Multiply(x=w197, y="Gain Mode 1") -> (x*y=w204:dbl)
            n67 = In Range and Coerce(upper limit=200.0, x=w204, lower limit=-200.0) -> (coerced(x)=→"duty":dbl)  [unwired: 1 out]
            n68 = call <vilib>:"Set Duty Cycle and Frequency.vi"("error in (no error)"=w198, "Frequency (Hz)"=w191, "Duty Cycle (0-1)"=w192, "PWM Ref In"=w212) -> ("error out"=w210:errorcluster)  [unwired: 5 in, 1 out]
            n69 = call <vilib>:"Set Duty Cycle and Frequency.vi"("error in (no error)"=w198, "Frequency (Hz)"=w189, "Duty Cycle (0-1)"=w190, "PWM Ref In"=w211) -> ("error out"=w209:errorcluster)  [unwired: 5 in, 1 out]
          }
          frame 0 {
            w216 = 50.0 ("freq [Hz]")
            w218 = 50.0 ("freq [Hz]")
            # "Moving Up Ramp Mode"
            n70 = Unbundle By Name(w225) -> ("Left Motor\nLeft Motor\nright_motor"=w224:T16)
            n71 = Unbundle By Name(w225) -> ("Right Motor\nleft_motor"=w223:T16)
            n72 = call "ServotoPWM.vi"("freq [Hz]"=w216, "Duty In"=w214) -> ("Duty Cycle"=w217:dbl)  [unwired: 6 in, 2 out]
            n73 = call "ServotoPWM.vi"("freq [Hz]"=w218, "Duty In"=w215) -> ("Duty Cycle"=w219:dbl)  [unwired: 6 in, 2 out]
            n74 = call <vilib>:"Set Duty Cycle and Frequency.vi"("error in (no error)"=w220, "Frequency (Hz)"=w218, "Duty Cycle (0-1)"=w219, "PWM Ref In"=w224) -> ("error out"=w222:errorcluster)  [unwired: 5 in, 1 out]
            n75 = call <vilib>:"Set Duty Cycle and Frequency.vi"("error in (no error)"=w220, "Frequency (Hz)"=w216, "Duty Cycle (0-1)"=w217, "PWM Ref In"=w223) -> ("error out"=w221:errorcluster)  [unwired: 5 in, 1 out]
          }
          frame 3, Default {
            w228 = 50.0 ("freq [Hz]")
            w230 = 50.0 ("freq [Hz]")
            # "Moving Up Ramp Mode"
            n76 = Unbundle By Name(w237) -> ("Left Motor\nLeft Motor\nright_motor"=w236:T16)
            n77 = Unbundle By Name(w237) -> ("Right Motor\nleft_motor"=w235:T16)
            n78 = call "ServotoPWM.vi"("freq [Hz]"=w228, "Duty In"=0.0) -> ("Duty Cycle"=w229:dbl)  [unwired: 6 in, 2 out]
            n79 = call "ServotoPWM.vi"("freq [Hz]"=w230, "Duty In"=0.0) -> ("Duty Cycle"=w231:dbl)  [unwired: 6 in, 2 out]
            n80 = call <vilib>:"Set Duty Cycle and Frequency.vi"("error in (no error)"=w232, "Frequency (Hz)"=w230, "Duty Cycle (0-1)"=w231, "PWM Ref In"=w236) -> ("error out"=w234:errorcluster)  [unwired: 5 in, 1 out]
            n81 = call <vilib>:"Set Duty Cycle and Frequency.vi"("error in (no error)"=w232, "Frequency (Hz)"=w228, "Duty Cycle (0-1)"=w229, "PWM Ref In"=w235) -> ("error out"=w233:errorcluster)  [unwired: 5 in, 1 out]
          }
          frame 2 {
            w254 = 0.95 ("Saturation U")
            w245 = 50.0 ("freq [Hz]")
            w246 = 50.0 ("freq [Hz]")
            # "Moving Down Ramp Mode"
            n82 = local read "Back Right"() -> (w261:dbl)
            n83 = local read "Back Left"() -> (w259:dbl)
            n84 = local read "duty 2"() -> (w250:dbl)
            n85 = local read "duty 2"() -> (w248:dbl)
            n86 = Subtract(x=w247, y=w248) -> (x-y=w243:dbl)
            n87 = Add(x=w249, y=w250) -> (x+y=w242:dbl)
            n88 = Subtract(x=w261, y=w259) -> (x-y=w260:dbl)
            n89 = Negate(x=w242) -> (-x=w241:dbl)
            "R_DC 2" <- w241
            n90 = Negate(x=w243) -> (-x=w244:dbl)
            "L_DC 2" <- w244
            n91 = call "contPIDantiWindupSubVI.vi"("Saturation M"=w254, "Saturation U"=w254, "PID Gains"="moving down ramp gainz", "Position"=w260, "Reference"=0.0) -> ("control"=w251:dbl)  [unwired: 6 in]
            "PID Output 2" <- w251
            n92 = Unbundle By Name(w267) -> ("Left Motor\nLeft Motor\nright_motor"=w266:T16)
            n93 = Unbundle By Name(w267) -> ("Right Motor\nleft_motor"=w265:T16)
            n94 = call "ServotoPWM.vi"("freq [Hz]"=w245, "Duty In"=w241) -> ("Duty Cycle"=w239:dbl)  [unwired: 6 in, 2 out]
            "Right Duty Cycle" <- w239
            n95 = call "ServotoPWM.vi"("freq [Hz]"=w246, "Duty In"=w244) -> ("Duty Cycle"=w238:dbl)  [unwired: 6 in, 2 out]
            "Left Duty Cycle" <- w238
            n96 = Multiply(x=w251, y="Gain Mode 2") -> (x*y=w258:dbl)
            n97 = In Range and Coerce(upper limit=200.0, x=w258, lower limit=-200.0) -> (coerced(x)=→"duty 2":dbl)  [unwired: 1 out]
            n98 = call <vilib>:"Set Duty Cycle and Frequency.vi"("error in (no error)"=w252, "Frequency (Hz)"=w245, "Duty Cycle (0-1)"=w239, "PWM Ref In"=w265) -> ("error out"=w263:errorcluster)  [unwired: 5 in, 1 out]
            n99 = call <vilib>:"Set Duty Cycle and Frequency.vi"("error in (no error)"=w252, "Frequency (Hz)"=w246, "Duty Cycle (0-1)"=w238, "PWM Ref In"=w266) -> ("error out"=w264:errorcluster)  [unwired: 5 in, 1 out]
          }
        }
        n100 = Unbundle By Name(w134) -> ("Windup"=w137:T16)
        n101 = call "ServotoPWMPulseWidth.vi"("freq [Hz]"=50.0, "Pulse Width"=w142) -> ("Duty Cycle"=w135:dbl)  [unwired: 6 in, 2 out]
        n102 = call <vilib>:"Set Duty Cycle and Frequency.vi"("error in (no error)"=w140, "Frequency (Hz)"=50.0, "Duty Cycle (0-1)"=w135, "PWM Ref In"=w137) -> ("error out"=w141:errorcluster)  [unwired: 5 in, 1 out]
        n103 = local read "Emergency Stop"() -> (w185:bool)
        n104 = Merge Errors(w125) -> (w133:errorcluster)
        n105 = node-c288() -> ()  [unwired: 1 in, 1 out]
        n106 = Merge Errors(w141, w140, w151, w150, w133) -> (w161:errorcluster)
      }
      n107 = flat-sequence {
        tunnel: [w88] -> w67
        tunnel: w63 -> [w87]
        tunnel: w62 -> [w85]
        tunnel: [w85] -> w61
        tunnel: w59 -> [w84]
        tunnel: [w84] -> w60
        tunnel: w67 -> [w99]
        tunnel: [w97] -> w64
        tunnel: w61 -> [w94]
        tunnel: w60 -> [w93]
        tunnel: [w92] -> w57
        frame #0 {
          # "Emergency Stop Interrupt"
          n108 = xnode "Invoke Method"("FPGA VI Reference In"=w87, "IRQ Number(s)"=0, "Timeout (ms)"=-1) -> ("FPGA VI Reference Out"=w91:refnum<k20>, "IRQ(s) Asserted"=w86:i32)  [unwired: 1 in, 2 out]
          n109 = xnode "Invoke Method"("FPGA VI Reference In"=w91, "IRQ Number(s)"=w86) -> ("FPGA VI Reference Out"=w88:refnum<k20>)  [unwired: 1 in, 1 out]
        }
        frame #1 {
          # "Turn Off All\nProcesses Here"
          n110 = for {
            N: 20 -> [_]
            tunnel: w99 -> [w118]
            tunnel: [w118] -> w97
            tunnel: w94 -> [w114]
            tunnel: [w114] -> _
            tunnel: w93 -> [w116]
            tunnel: [w113] -> w92
            w104 = 50.0 ("Frequency (Hz)")
            w108 = 50.0 ("Frequency (Hz)")
            n111 = Unbundle By Name(w114) -> ("LED Ref"=w117:T4)
            n112 = Wait (ms)(milliseconds to wait=u32 100) -> ()  [unwired: 1 out]
            n113 = Unbundle By Name(w114) -> ("Left Motor\nLeft Motor\nright_motor"=w103:T16)
            n114 = call <vilib>:"Write.vi"("error in (no error)"=w116, "Values"=bool[] [FALSE, FALSE, FALSE, FALSE], "DIO Ref In"=w117) -> ()  [unwired: 6 in, 2 out]
            n115 = call "ServotoPWMPulseWidth.vi"("freq [Hz]"=w104, "Pulse Width"=1500.0) -> ("Duty Cycle"=w105:dbl)  [unwired: 6 in, 2 out]
            n116 = call <vilib>:"Set Duty Cycle and Frequency.vi"("Frequency (Hz)"=w104, "Duty Cycle (0-1)"=w105, "PWM Ref In"=w103) -> ()  [unwired: 6 in, 2 out]
            n117 = Unbundle By Name(w114) -> ("Right Motor\nleft_motor"=w102:T16)
            n118 = call "ServotoPWMPulseWidth.vi"("freq [Hz]"=w108, "Pulse Width"=1500.0) -> ("Duty Cycle"=w109:dbl)  [unwired: 6 in, 2 out]
            n119 = call <vilib>:"Set Duty Cycle and Frequency.vi"("Frequency (Hz)"=w108, "Duty Cycle (0-1)"=w109, "PWM Ref In"=w102) -> ()  [unwired: 6 in, 2 out]
            n120 = Unbundle By Name(w114) -> ("Windup"=w111:T16)
            n121 = call <vilib>:"Set Duty Cycle and Frequency.vi"("Frequency (Hz)"=50.0, "Duty Cycle (0-1)"=1525.0, "PWM Ref In"=w111) -> ("error out"=w113:errorcluster)  [unwired: 6 in, 1 out]
            "Emergency Stop" <- TRUE ("Emergency Stop")
          }
          n122 = property on="Black Box" class="WFChart (strict)"() -> ("History Data"=w96:T25)  [unwired: 2 in, 2 out]
          n123 = for {
            tunnel: w96 -> [w101] mode=indexing
            tunnel: [w100] -> w95 mode=indexing
            n124 = Cluster To Array(cluster=w101) -> (array=w100:dbl[])
          }
          "Black Box Array" <- w95
        }
      }
      n125 = node-c288() -> (w66:T20)  [unwired: 4 in]
      n126 = timed-loop {
        timing: w66 -> [_]
        timing-out: [_] -> w65
        stop <- w77 stop-if-true
        # "Black Box Code"
        n127 = node-c288() -> ()  [unwired: 1 in, 1 out]
        n128 = local read "Button Num"() -> (w72:u32)
        n129 = local read "Button Num"() -> (w70:u32)
        n130 = local read "Button Num"() -> (w71:u32)
        n131 = To Double Precision Float(number=w72) -> (double precision float=w73:dbl)
        n132 = To Double Precision Float(number=w71) -> (double precision float=w75:dbl)
        n133 = To Double Precision Float(number=w70) -> (double precision float=w76:dbl)
        n134 = Build Array(w73, w75, w76) -> (w74:dbl[])
        n135 = local read "Emergency Stop"() -> (w77:bool)
        n136 = disable-structure shown="Disabled" {
          disable-tunnel: w74 -> [w79 _]
          frame Disabled {
            n137 = Array To Cluster(array=w79) -> (cluster=→"Black Box":T1)
          }
          frame Enabled {
          }
        }
        n138 = node-c288() -> ()  [unwired: 1 in, 1 out]
      }
      n139 = node-c288(w65) -> ()  [unwired: 1 out]
      n140 = node-c288(w68) -> ()  [unwired: 1 out]
    }
    frame #2 {
      n141 = Unbundle By Name(w404) -> ("Button Ref"=w403:T4, "LED Ref"=w402:T4, "Front_Right"=w396:T11, "Front_Left"=w394:T11, "Back_Right"=w393:T11, "Front_Center\nBI Ref 1"=w392:T11, "Back_Left\nBI Ref 2"=w391:T11, "Windup"=w386:T16, "Platform_S\nPlatform_S\nContinuous Servo"=w384:T16, "Left Motor\nLeft Motor\nright_motor"=w378:T16, "Right Motor\nleft_motor"=w381:T16)
      n142 = call <vilib>:"Close.vi"("error in (no error)"=w379, "DIO Ref In"=w403) -> ("error out"=w401:errorcluster)  [unwired: 9 in]
      n143 = call <vilib>:"Close.vi"("error in (no error)"=w379, "DIO Ref In"=w402) -> ("error out"=w400:errorcluster)  [unwired: 9 in]
      n144 = call <vilib>:"Close.vi"("error in (no error)"=w379, "AI Ref In"=w396) -> ("error out"=w395:errorcluster)  [unwired: 9 in]
      n145 = call <vilib>:"Close.vi"("error in (no error)"=w379, "AI Ref In"=w394) -> ("error out"=w390:errorcluster)  [unwired: 9 in]
      n146 = call <vilib>:"Close.vi"("error in (no error)"=w379, "PWM Ref In"=w384) -> ("error out"=w383:errorcluster)  [unwired: 9 in]
      n147 = call <vilib>:"Close.vi"("error in (no error)"=w379, "AI Ref In"=w393) -> ("error out"=w389:errorcluster)  [unwired: 9 in]
      n148 = call <vilib>:"Close.vi"("error in (no error)"=w379, "AI Ref In"=w392) -> ("error out"=w388:errorcluster)  [unwired: 9 in]
      n149 = call <vilib>:"Close.vi"("error in (no error)"=w379, "AI Ref In"=w391) -> ("error out"=w387:errorcluster)  [unwired: 9 in]
      n150 = call <vilib>:"Close.vi"("error in (no error)"=w379, "PWM Ref In"=w386) -> ("error out"=w385:errorcluster)  [unwired: 9 in]
      n151 = call <vilib>:"Close.vi"("error in (no error)"=w379, "PWM Ref In"=w378) -> ("error out"=w382:errorcluster)  [unwired: 9 in]
      n152 = call <vilib>:"Close.vi"("error in (no error)"=w379, "PWM Ref In"=w381) -> ("error out"=w380:errorcluster)  [unwired: 9 in]
      n153 = Merge Errors(w401, w400, w397, w395, w390, w389, w388, w387, w385, w383, w382, w380) -> (w399:errorcluster)
      n154 = xnode "Close FPGA VI Reference"("FPGA VI Reference In"=w405, "error in"=w399) -> ("error out"=w398:errorcluster)
      n155 = call <vilib>:"Simple Error Handler.vi"("error in (no error)"=w398) -> ()  [unwired: 4 in, 5 out]
    }
  }
